vi "Get_OwningVIPanel.vi"(8 "error in (no error)":errorcluster, 10 "Control Label":string, 11 "CtlLookup In":T1) -> (0 "error out":errorcluster, 1 "Owning VI":refnum<vi>, 2 "Front Panel":refnum<vi>, 3 "CtlLookup Out":T1)   [LabVIEW 2020, in "CtlReferences.lvlib" / "CtlReferences.lvclass"]
doc: "Gets the owning pane and panel of the specified control"
uses:
  CtlReferences.lvclass
  TypeDefs/CtlLookup.ctl
  CtlReferences.lvclass/CtlReferences.ctl
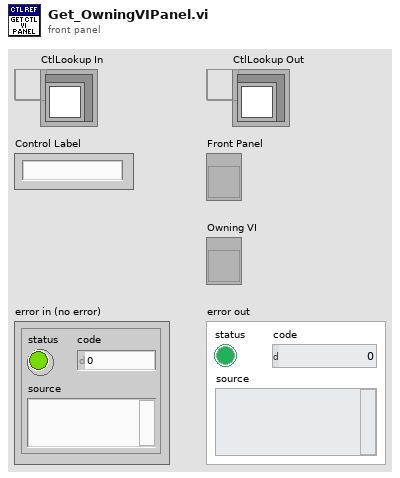
[diagram p1: front panel]
types:
  T1 = typedef "CtlReferences.lvlib/CtlReferences.lvclass/CtlLookup.ctl" = refnum<data-value>
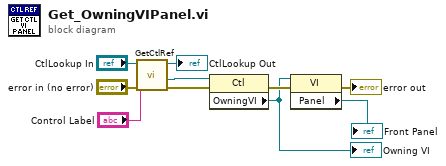
[diagram p0: block diagram]
diagram:
  n1 = call "GetCtlRef.vi"("Error in"="error in (no error)", "CtlName In"="Control Label", "CtlLookup In"="CtlLookup In") -> ("error out"=w8:errorcluster, "CtlRef"=w7:refnum<vi>, "CtlLookup Out"=→"CtlLookup Out":T1)  [unwired: 5 in, 1 out]
  n2 = property class="Ctl"(reference=w7, error in=w8) -> (error out=w10:errorcluster, "OwningVI"=w9:refnum<vi>)  [unwired: 1 out]
  "Owning VI" <- w9
  n3 = property class="VI"(reference=w9, error in=w10) -> (error out=→"error out":errorcluster, "Panel"=→"Front Panel":refnum<vi>)  [unwired: 1 out]
